vi "Constants.vi"() -> ()   [LabVIEW 2016, in "UDP Sender Shared.lvlib"]
doc: "Use this Global VI to access the GUIDs assigned to the page resources of the Custom Device."
uses:
  UDP Sender Shared.lvlib
panel:
  in  "Tab Control":enum32{"GUIDS", "Constants", "Properties"}(tab)=enum."Properties"
  in  "UDP Sender":string="51b5d3ac-e502-4eda-8223-78fc965f9b7d"
  in  "Destination Port":string="Destination Port"
  in  "Destination Address":string="Destination Address"
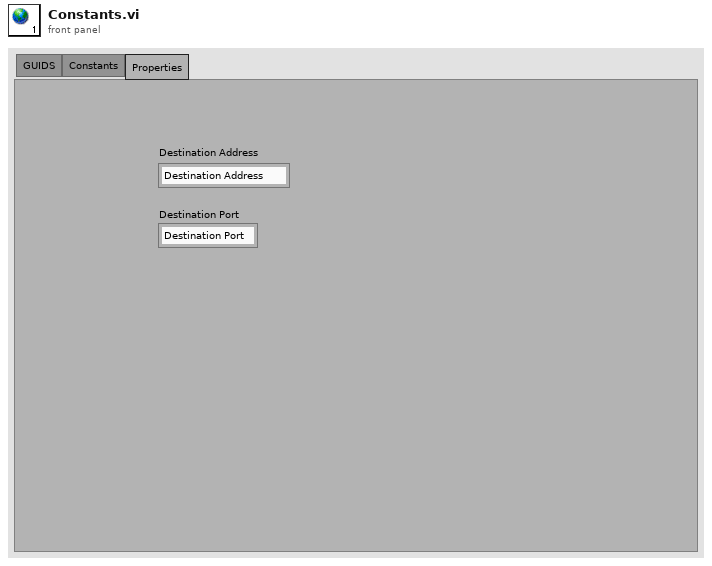
[diagram p1: front panel]
diagram:
